vi "GetWaveformByName.vi"(8 "error in (no error)":errorcluster, 10 "Channel Name":string, 11 "Acq Waveforms":waveform(sgl)[](array[waveform])) -> (0 "error out":errorcluster, 1 "Waveform":waveform(sgl), 2 "Found?":bool, 3 "Acq Waveforms Out":waveform(sgl)[](array[waveform]))   [LabVIEW 2017]
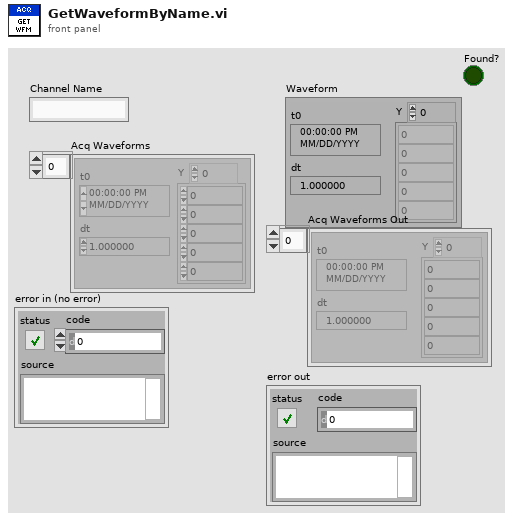
[diagram p1: front panel]
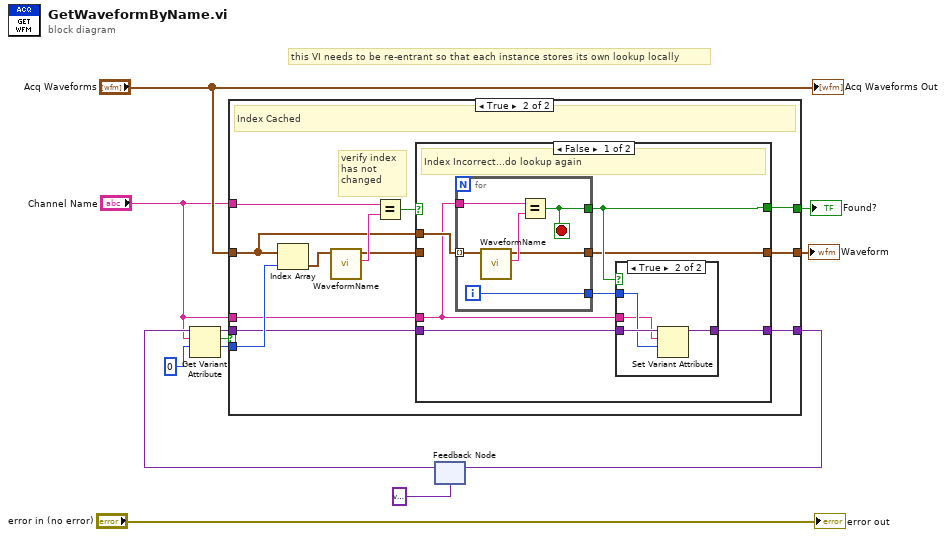
[diagram p0: block diagram]
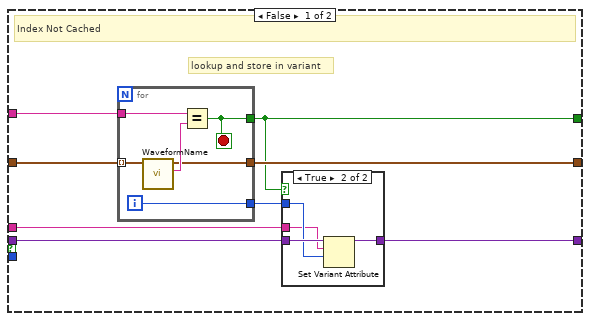
[diagram p2: hidden frame]
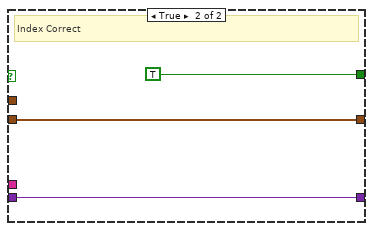
[diagram p5: hidden frame]
diagram:
  # "this VI needs to be re-entrant so that each instance stores its own lookup locally"
  n1 = feedback #1(variant) -> (w7:variant)
  n2 = Get Variant Attribute(Variant=w7, name="Channel Name", default value (empty Variant)=0) -> (duplicate Variant=w4:variant, found=w5:bool, value=w3:i32)  [unwired: 1 in, 1 out]
  n3 = case shown="True" w5 {
    tunnel: [w20 w37] -> w12
    tunnel: "Acq Waveforms" -> [w19 w32]
    tunnel: [w17 w36] -> w10
    tunnel: "Channel Name" -> [w18 w40]
    tunnel: w4 -> [w15 w35]
    tunnel: w3 -> [_ w43]
    tunnel: "Channel Name" -> [w14 w33]
    tunnel: [w13 w34] -> w1
    frame False {
      # "lookup and store in variant"
      # "Index Not Cached"
      n4 = for {
        tunnel: w19 -> [w31] mode=indexing
        tunnel: w18 -> [w30]
        tunnel: [w27] -> w20
        tunnel: [w29] -> w17
        tunnel: [w26] -> w16
        i -> [w26]
        stop <- w29 stop-if-true
        n5 = call <vilib>:"WaveformName.vi"("signal in"=w31) -> ("name"=w28:string, "signal out"=w27:waveform(sgl))  [unwired: 9 in]
        n6 = Equal?(x=w30, y=w28) -> (x = y?=w29:bool)
      }
      n7 = case shown="True" w17 {
        tunnel: w16 -> [_ w24]
        tunnel: w15 -> [w21 w25]
        tunnel: w14 -> [_ w23]
        tunnel: [w21 w22] -> w13
        frame False {
        }
        frame True {
          n8 = Set Variant Attribute(Variant=w25, name=w23, value=w24) -> (Variant out=w22:variant)  [unwired: 1 in, 2 out]
        }
      }
    }
    frame True {
      # "verify index has not changed"
      # "Index Cached"
      n9 = Index Array(array=w32, index=w43) -> (element=w42:waveform(sgl))
      n10 = call <vilib>:"WaveformName.vi"("signal in"=w42) -> ("name"=w41:string, "signal out"=w38:waveform(sgl))  [unwired: 9 in]
      n11 = Equal?(x=w40, y=w41) -> (x = y?=w39:bool)
      n12 = case shown="False" w39 {
        tunnel: w38 -> [_ w64]
        tunnel: [w44 w64] -> w37
        tunnel: [w45 TRUE] -> w36
        tunnel: [w48 w62] -> w34
        tunnel: w35 -> [w49 w62]
        tunnel: w33 -> [w46 _]
        tunnel: w32 -> [w47 _]
        frame False {
          # "Index Incorrect...do lookup again"
          n13 = for {
            tunnel: w47 -> [w61] mode=indexing
            tunnel: w46 -> [w60]
            tunnel: [w57] -> w44
            tunnel: [w59] -> w45
            tunnel: [w56] -> w50
            i -> [w56]
            stop <- w59 stop-if-true
            n14 = call <vilib>:"WaveformName.vi"("signal in"=w61) -> ("name"=w58:string, "signal out"=w57:waveform(sgl))  [unwired: 9 in]
            n15 = Equal?(x=w60, y=w58) -> (x = y?=w59:bool)
          }
          n16 = case shown="True" w45 {
            tunnel: w50 -> [_ w54]
            tunnel: w49 -> [w51 w55]
            tunnel: w46 -> [_ w53]
            tunnel: [w51 w52] -> w48
            frame False {
            }
            frame True {
              n17 = Set Variant Attribute(Variant=w55, name=w53, value=w54) -> (Variant out=w52:variant)  [unwired: 1 in, 2 out]
            }
          }
        }
        frame True {
          # "Index Correct"
        }
      }
    }
  }
  "Waveform" <- w12
  "Found?" <- w10
  n18 = feedback-in #1(w1) -> ()
  "Acq Waveforms Out" <- "Acq Waveforms"
  "error out" <- "error in (no error)"
